vi "_PC_Pub_FM writeData.vi"(8 "error in (no error)":errorcluster, 10 "element":waveform(sgl), 11 "FM in":refnum<class "FM.lvclass">) -> (0 "error out":errorcluster, 3 "FM out":refnum<class "FM.lvclass">)   [LabVIEW 2018, in "FM.lvclass"]
uses:
  FM.lvclass
  FM.lvclass/FM.ctl
  TDMSAdv/TDMSAdv writeOfString.vi
  TDMSAdv/TDMSAdv writeOfI16.vi
  TDMSAdv/TDMSAdv writeOfDBL.vi
  TDMSAdv/TDMSAdv writeOfSGL.vi
  TDMSAdv.lvclass
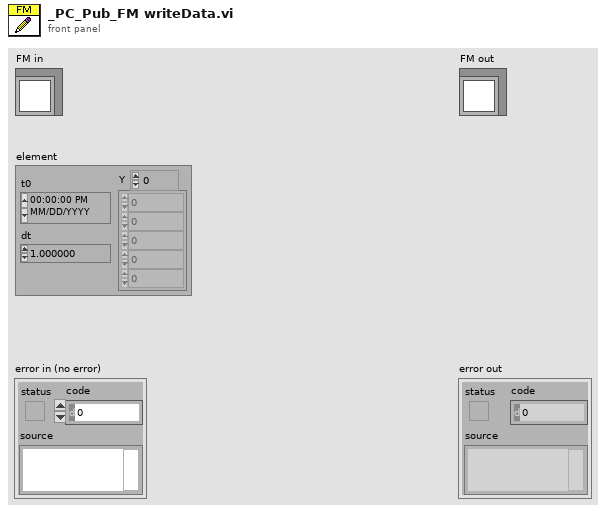
[diagram p1: front panel]
types:
  T1 = cluster{"attrData":string, "mzRange":string, "dt":dbl, "yData":sgl[], "dataTime":timestamp}
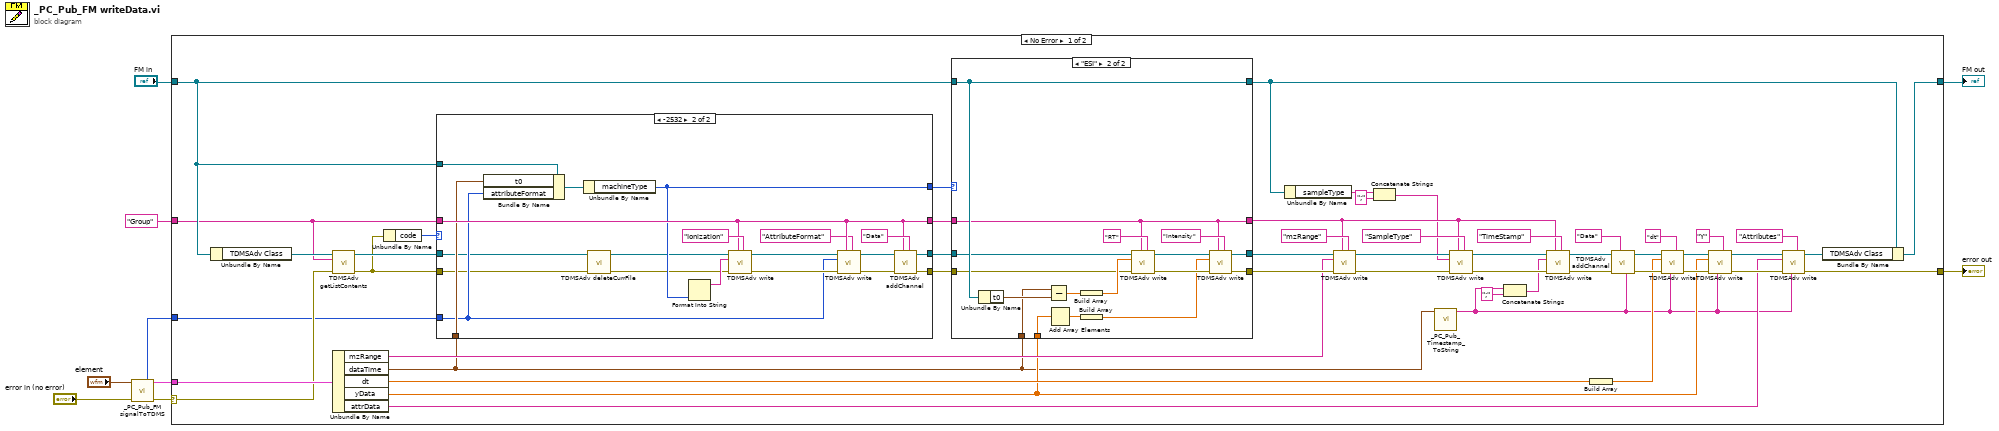
[diagram p0: block diagram]
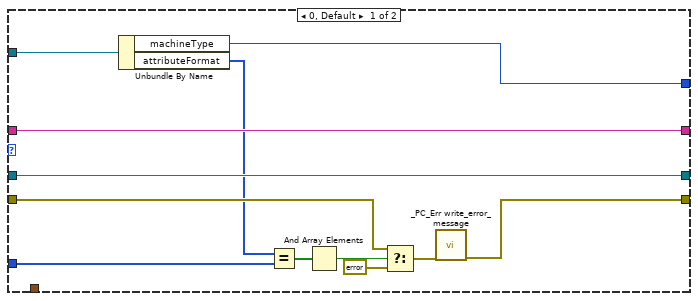
[diagram p2: hidden frame]
diagram:
  n1 = call "_PC_Pub_FM signalToTDMS.vi"("error in (no error)"="error in (no error)", "SignalData"="element") -> ("error out"=w3:errorcluster, "dataParam"=w4:T1, "attrType"=w5:i16[])  [unwired: 7 in]
  n2 = case shown="No Error" w3 {
    selector: w3 -> [w23 w115]
    tunnel: [w14 w115] -> w9
    tunnel: [w37 w114] -> w7
    tunnel: "FM in" -> [w22 w114]
    tunnel: "Group" ("group name (Untitled)") -> [w10 _]
    tunnel: w4 -> [w33 _]
    tunnel: w5 -> [w18 _]
    frame No Error {
      n3 = Unbundle By Name(w22) -> ("TDMSAdv Class"=w24:refnum<class "TDMSAdv.lvclass">)
      n4 = call "TDMSAdv getListContents.vi"("error in (no error)"=w23, "group name"=w10, "TDMSAdv in"=w24) -> ("error out"=w11:errorcluster, "TDMSAdv out"=w16:refnum<class "TDMSAdv.lvclass">)  [unwired: 6 in, 1 out]
      n5 = Unbundle By Name(w33) -> ("mzRange"=w29:string, "dataTime"=w17:timestamp, "dt"=w32:dbl, "yData"=w28:sgl[], "attrData"=w30:string)
      n6 = Unbundle By Name(w11) -> ("code"=w12:i32)
      n7 = case shown="-2532" w12 {
        tunnel: w16 -> [w70 w76]
        tunnel: w10 -> [w72 w87]
        tunnel: w11 -> [w67 w74]
        tunnel: [w64 w90] -> w19
        tunnel: [w70 w91] -> w20
        tunnel: [w72 w87] -> w21
        tunnel: w18 -> [w71 w77]
        tunnel: w17 -> [_ w78]
        tunnel: w22 -> [w63 w80]
        tunnel: [w61 w82] -> w15
        frame 0, Default {
          n8 = Unbundle By Name(w63) -> ("machineType"=w61:enum16{"MALDI", "ESI"}, "attributeFormat"=w62:i16[])
          n9 = Equal?(x=w62, y=w71) -> (x = y?=w69:bool[])
          n10 = And Array Elements(Boolean array=w69) -> (logical AND=w68:bool)
          n11 = Select(t=w67, s=w68, f=errorcluster {"status"=TRUE, "code"=6001, "source"="Attribute Format Different"}) -> (s? t:f=w65:errorcluster)
          n12 = call "_PC_Err write_error_message.vi"("error in"=w65) -> ("error out"=w64:errorcluster)  [unwired: 10 in]
        }
        frame -2532 {
          n13 = Bundle By Name(cluster=w80, "t0"=w78, "attributeFormat"=w77) -> (w79:refnum<class "FM.lvclass">)
          n14 = Unbundle By Name(w79) -> ("machineType"=w82:enum16{"MALDI", "ESI"})
          n15 = call "TDMSAdv deleteCurrFile .vi"("error in (no error)"=w74, "TDMSAdv in"=w76) -> ("error out"=w73:errorcluster, "TDMSAdv out"=w75:refnum<class "TDMSAdv.lvclass">)  [unwired: 8 in]
          n16 = Format Into String(w82) -> (resulting string=w81:string)  [unwired: 3 in, 1 out]
          n17 = call-poly "TDMSAdv write.vi"("channel name"="Ionization", "group name (Untitled)"=w87, "error in (no error)"=w73, "dataArray"=w81, "TDMSAdv in"=w75) -> ("error out"=w85:errorcluster, "TDMSAdv out"=w88:refnum<class "TDMSAdv.lvclass">)  [unwired: 5 in]
          n18 = call-poly "TDMSAdv write.vi"("channel name"="AttributeFormat", "group name (Untitled)"=w87, "error in (no error)"=w85, "dataArray"=w77, "TDMSAdv in"=w88) -> ("error out"=w83:errorcluster, "TDMSAdv out"=w84:refnum<class "TDMSAdv.lvclass">)  [unwired: 5 in]
          n19 = call "TDMSAdv addChannel.vi"("channel name"="Data", "group name (Untitled)"=w87, "error in (no error)"=w83, "TDMSAdv in"=w84) -> ("error out"=w90:errorcluster, "TDMSAdv out"=w91:refnum<class "TDMSAdv.lvclass">)  [unwired: 6 in]
        }
      }
      n20 = case shown="\"ESI\"" w15 {
        tunnel: [w96 w102] -> w38
        tunnel: w22 -> [w96 w102]
        tunnel: w21 -> [w95 w99]
        tunnel: w19 -> [w93 w100]
        tunnel: [w95 w99] -> w55
        tunnel: [w94 w104] -> w52
        tunnel: [w93 w103] -> w51
        tunnel: w20 -> [w94 w101]
        tunnel: w28 -> [_ w98]
        tunnel: w17 -> [_ w97]
        frame "MALDI", Default {
        }
        frame "ESI" {
          n21 = Unbundle By Name(w102) -> ("t0"=w109:timestamp)
          n22 = Subtract(x=w97, y=w109) -> (x-y=w108:dbl)
          n23 = Add Array Elements(numeric array=w98) -> (sum=w106:sgl)
          n24 = Build Array(w108) -> (w107:dbl[])
          n25 = Build Array(w106) -> (w105:sgl[])
          n26 = call-poly "TDMSAdv write.vi"("channel name"="RT", "group name (Untitled)"=w99, "error in (no error)"=w100, "dataArray"=w107, "TDMSAdv in"=w101) -> ("error out"=w110:errorcluster, "TDMSAdv out"=w111:refnum<class "TDMSAdv.lvclass">)  [unwired: 5 in]
          n27 = call-poly "TDMSAdv write.vi"("channel name"="Intensity", "group name (Untitled)"=w99, "error in (no error)"=w110, "dataArray"=w105, "TDMSAdv in"=w111) -> ("error out"=w103:errorcluster, "TDMSAdv out"=w104:refnum<class "TDMSAdv.lvclass">)  [unwired: 5 in]
        }
      }
      n28 = Unbundle By Name(w38) -> ("sampleType"=w36:string)
      n29 = call-poly "TDMSAdv write.vi"("channel name"="mzRange", "group name (Untitled)"=w55, "error in (no error)"=w51, "dataArray"=w29, "TDMSAdv in"=w52) -> ("error out"=w53:errorcluster, "TDMSAdv out"=w54:refnum<class "TDMSAdv.lvclass">)  [unwired: 5 in]
      n30 = Concatenate Strings(w36, ";" ("string")) -> (w34:string)
      n31 = call "_PC_Pub_Timestamp_ToString.vi"("Timestamp"=w17) -> ("Timestring"=w26:string)  [unwired: 9 in, 1 out]
      n32 = call-poly "TDMSAdv write.vi"("channel name"="SampleType", "group name (Untitled)"=w55, "error in (no error)"=w53, "dataArray"=w34, "TDMSAdv in"=w54) -> ("error out"=w58:errorcluster, "TDMSAdv out"=w57:refnum<class "TDMSAdv.lvclass">)  [unwired: 5 in]
      n33 = Concatenate Strings(w26, ";" ("string")) -> (w25:string)
      n34 = call-poly "TDMSAdv write.vi"("channel name"="TimeStamp", "group name (Untitled)"=w55, "error in (no error)"=w58, "dataArray"=w25, "TDMSAdv in"=w57) -> ("error out"=w41:errorcluster, "TDMSAdv out"=w42:refnum<class "TDMSAdv.lvclass">)  [unwired: 5 in]
      n35 = Build Array(w32) -> (w31:dbl[])
      n36 = call "TDMSAdv addChannel.vi"("channel name"=w26, "group name (Untitled)"="Data" ("channel name"), "error in (no error)"=w41, "TDMSAdv in"=w42) -> ("error out"=w39:errorcluster, "TDMSAdv out"=w40:refnum<class "TDMSAdv.lvclass">)  [unwired: 6 in]
      n37 = call-poly "TDMSAdv write.vi"("channel name"="dt", "group name (Untitled)"=w26, "error in (no error)"=w39, "dataArray"=w31, "TDMSAdv in"=w40) -> ("error out"=w44:errorcluster, "TDMSAdv out"=w45:refnum<class "TDMSAdv.lvclass">)  [unwired: 5 in]
      n38 = call-poly "TDMSAdv write.vi"("channel name"="Y", "group name (Untitled)"=w26, "error in (no error)"=w44, "dataArray"=w28, "TDMSAdv in"=w45) -> ("error out"=w48:errorcluster, "TDMSAdv out"=w47:refnum<class "TDMSAdv.lvclass">)  [unwired: 5 in]
      n39 = call-poly "TDMSAdv write.vi"("channel name"="Attributes", "group name (Untitled)"=w26, "error in (no error)"=w48, "dataArray"=w30, "TDMSAdv in"=w47) -> ("error out"=w14:errorcluster, "TDMSAdv out"=w13:refnum<class "TDMSAdv.lvclass">)  [unwired: 5 in]
      n40 = Bundle By Name(cluster=w38, "TDMSAdv Class"=w13) -> (w37:refnum<class "FM.lvclass">)
    }
    frame Error {
    }
  }
  "error out" <- w9
  "FM out" <- w7
